vi "Road.vi"(1 "Road Width":i8, 2 "coordinate":T1, 3 "Map in":bool[][](array[boolean])) -> (0 "Map out":bool[][](array[boolean]))   [LabVIEW 2020]
uses:
  <vilib>/numeric/Random Number (Range) I64.vi
  <vilib>/numeric/sub_Random U32.vi
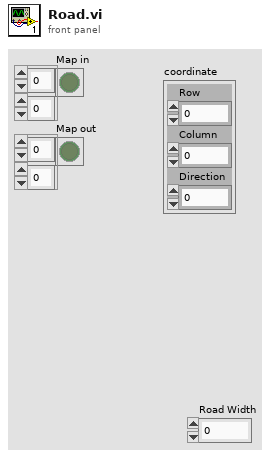
[diagram p1: front panel]
types:
  T1 = cluster{"Row":i32, "Column":i32, "Direction":i32}
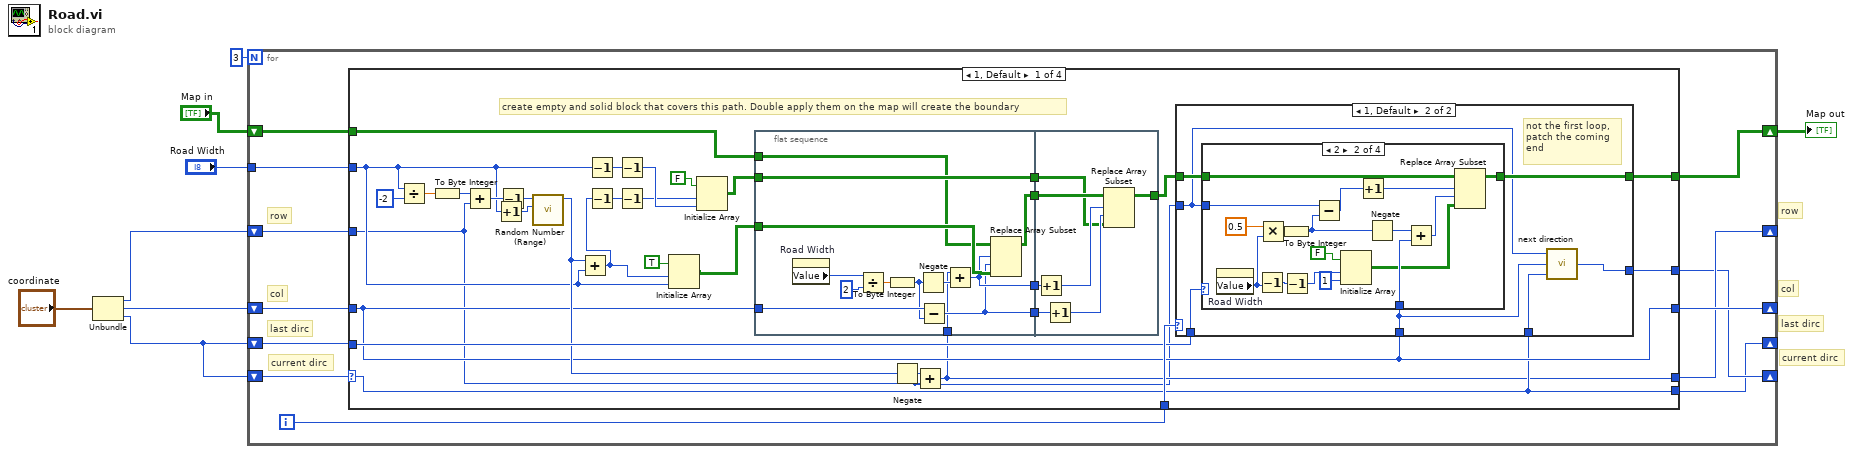
[diagram p0: block diagram]
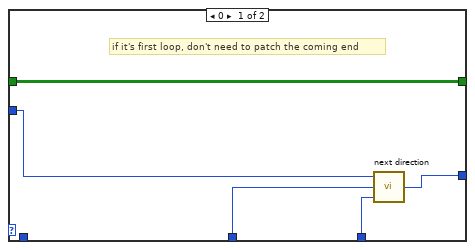
[diagram p2: hidden frame]
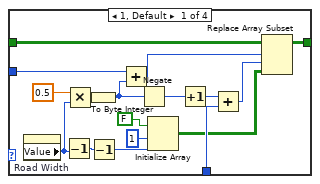
[diagram p3: hidden frame]
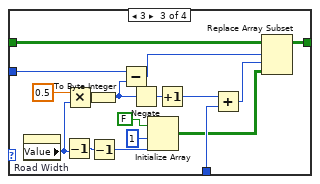
[diagram p4: hidden frame]
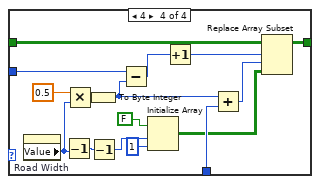
[diagram p5: hidden frame]
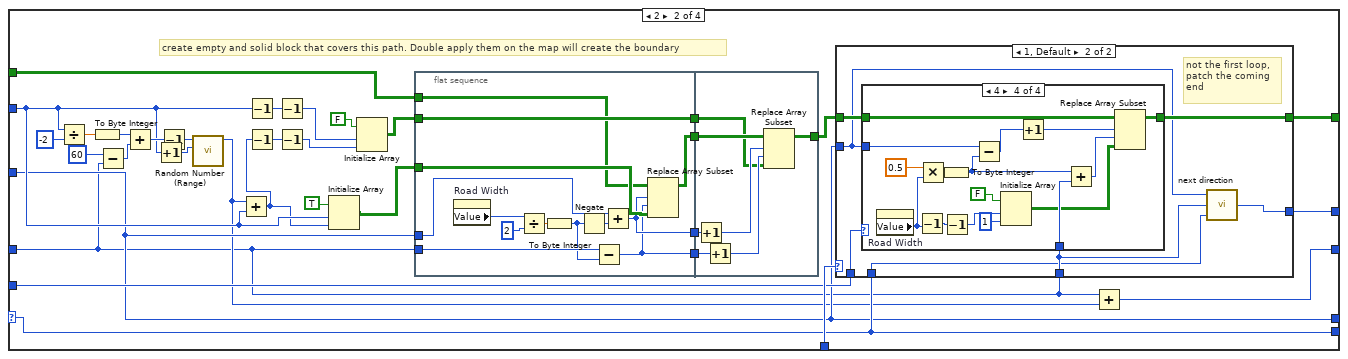
[diagram p6: hidden frame]
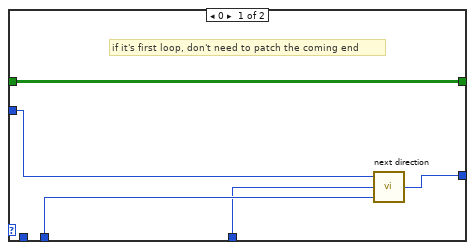
[diagram p7: hidden frame]
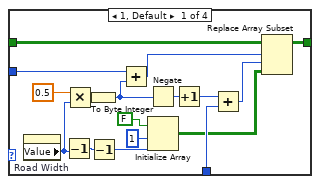
[diagram p8: hidden frame]
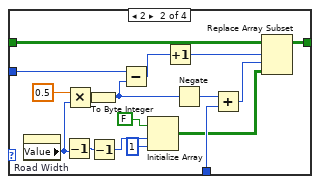
[diagram p9: hidden frame]
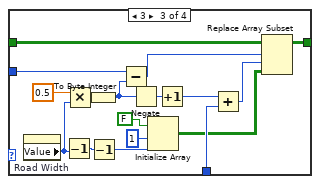
[diagram p10: hidden frame]
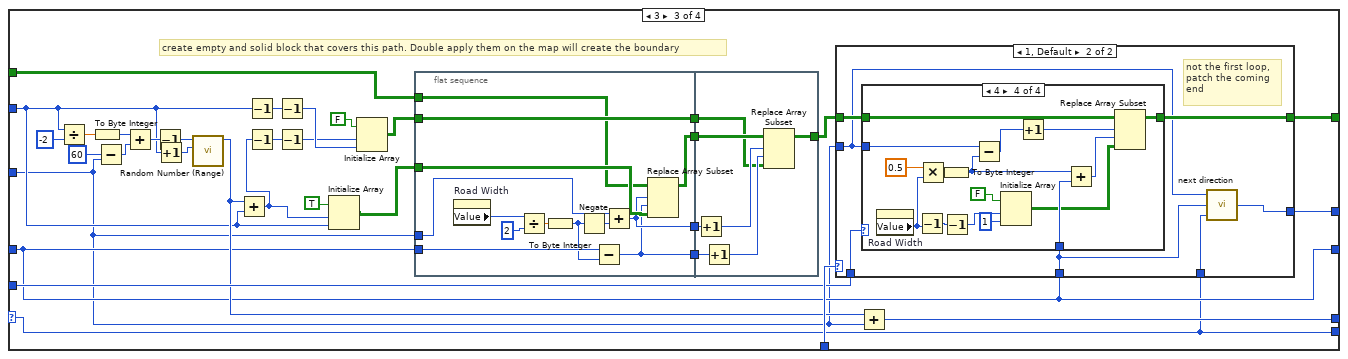
[diagram p11: hidden frame]
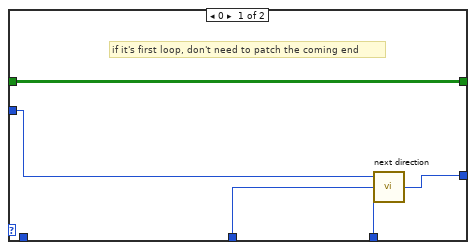
[diagram p12: hidden frame]
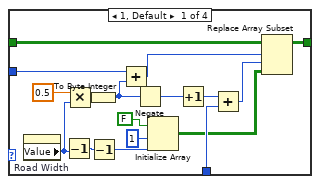
[diagram p13: hidden frame]
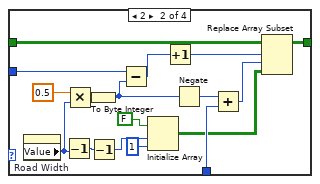
[diagram p14: hidden frame]
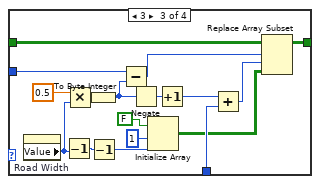
[diagram p15: hidden frame]
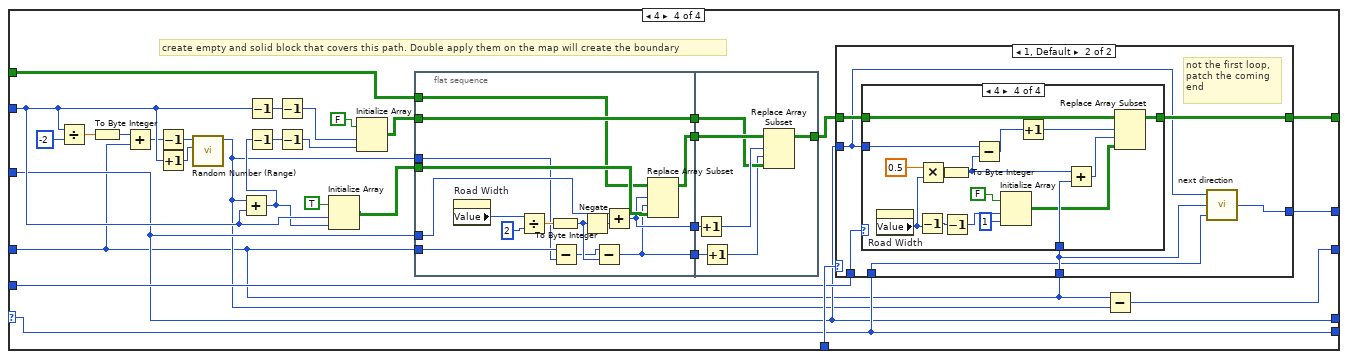
[diagram p16: hidden frame]
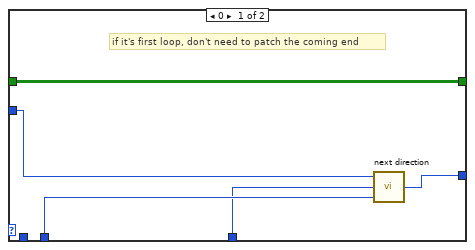
[diagram p17: hidden frame]
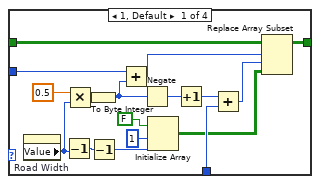
[diagram p18: hidden frame]
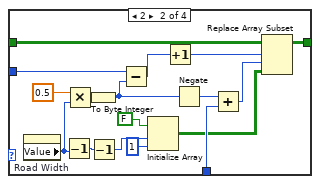
[diagram p19: hidden frame]
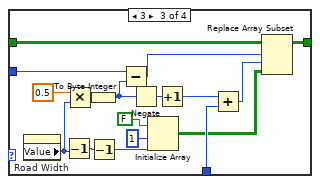
[diagram p20: hidden frame]
diagram:
  # "row"
  # "col"
  # "last dirc"
  # "current dirc"
  n1 = Unbundle("coordinate") -> ("Row"=w3:i32, "Column"=w2:i32, "Direction"=w1:i32)
  n2 = for {
    N: 3 -> [_]
    tunnel: "Road Width" -> [w19]
    shift-right: [w12] -> _
    shift-left: w1 -> [w20]
    shift-right: [w11] -> _
    shift-left: w1 -> [w14]
    shift-right: [w13] -> _
    shift-left: w3 -> [w10]
    shift-right: [w16] -> _
    shift-left: w2 -> [w18]
    shift-right: [w15] -> w5
    shift-left: "Map in" -> [w17]
    i -> [w9]
    # "row"
    # "col"
    # "last dirc"
    # "current dirc"
    n3 = case shown="1, Default" w20 {
      selector: w20 -> [w26 w163 w289 w427]
      tunnel: w19 -> [w30 w158 w294 w424]
      tunnel: w10 -> [w21 w155 w284 w419]
      tunnel: w18 -> [w29 w152 w293 w416]
      tunnel: w17 -> [w31 w166 w295 w430]
      tunnel: w9 -> [w52 w184 w316 w446]
      tunnel: [w22 w155 w292 w419] -> w13
      tunnel: [w29 w154 w293 w418] -> w16
      tunnel: [w51 w183 w315 w445] -> w15
      tunnel: w14 -> [w50 w182 w314 w444]
      tunnel: [w27 w164 w290 w428] -> w12
      tunnel: [w26 w163 w289 w427] -> w11
      frame 1, Default {
        # "create empty and solid block that covers this path. Double apply them on the map will create the boundary"
        n4 = Divide(x=w30, y=i8 -2) -> (x/y=w33:dbl)
        n5 = To Byte Integer(number=w33) -> (8bit integer=w34:i8)
        n6 = Add(x=w34, y=w21) -> (x+y=w35:i64)
        n7 = Increment(x=w30) -> (x+1=w36:i8)
        n8 = Decrement(x=w35) -> (x-1=w23:i64)
        n9 = call-poly <vilib>:"Random Number (Range).vi"("lower bound (-100)"=w36, "upper bound (100)"=w23) -> ("number"=w45:i64)  [unwired: 9 in]
        n10 = Add(x=w45, y=w30) -> (x+y=w24:i64)
        n11 = Decrement(x=w30) -> (x-1=w41:i8)
        n12 = Decrement(x=w24) -> (x-1=w39:i64)
        n13 = Decrement(x=w41) -> (x-1=w42:i8)
        n14 = Decrement(x=w39) -> (x-1=w40:i64)
        n15 = Initialize Array(TRUE, w24, w30) -> (w43:bool[][])
        n16 = Initialize Array(FALSE, w40, w42) -> (w44:bool[][])
        n17 = flat-sequence {
          tunnel: w29 -> [w63]
          tunnel: [w61] -> w49
          tunnel: w43 -> [w60]
          tunnel: [w59] -> w48
          tunnel: [w58] -> w47
          tunnel: w44 -> [w57]
          tunnel: [w57] -> w46
          tunnel: w31 -> [w56]
          tunnel: w22 -> [w53]
          tunnel: w49 -> [w72]
          tunnel: w48 -> [w71]
          tunnel: w47 -> [w69]
          tunnel: w46 -> [w67]
          tunnel: [w66] -> w28
          frame #0 {
            n18 = property on="Road Width" class="DigNum (strict)"() -> ("Value"=w55:i8)  [unwired: 2 in, 2 out]
            n19 = Divide(x=w55, y=i8 2) -> (x/y=w64:dbl)
            n20 = To Byte Integer(number=w64) -> (8bit integer=w62:i8)
            n21 = Negate(x=w62) -> (-x=w54:i8)
            n22 = Subtract(x=w63, y=w62) -> (x-y=w58:i64)
            n23 = Add(x=w53, y=w54) -> (x+y=w59:i64)
            n24 = Replace Array Subset(array=w56, new element=w60, index (row)=w59, index (col)=w58) -> (w61:bool[][])
          }
          frame #1 {
            n25 = Increment(x=w71) -> (x+1=w70:i64)
            n26 = Increment(x=w69) -> (x+1=w68:i64)
            n27 = Replace Array Subset(array=w72, new element=w67, index (row)=w70, index (col)=w68) -> (w66:bool[][])
          }
        }
        n28 = Negate(x=w45) -> (-x=w25:i64)
        n29 = Add(x=w25, y=w21) -> (x+y=w22:i64)
        n30 = case shown="1, Default" w52 {
          tunnel: [w77 w83] -> w51
          tunnel: w50 -> [_ w84]
          tunnel: w21 -> [w73 w81]
          tunnel: w29 -> [w75 w79]
          tunnel: w28 -> [w77 w82]
          tunnel: w26 -> [w76 w78]
          tunnel: [w74 w80] -> w27
          frame 0 {
            # "if it's first loop, don't need to patch the coming end"
            n31 = call "next direction.vi"("current direc"=w76, "col"=w75, "row"=w73) -> ("next direc"=w74:i32)
          }
          frame 1, Default {
            # "not the first loop,\npatch the coming\nend"
            n32 = case shown="2" w84 {
              tunnel: w81 -> [w94 w113 w128 w146]
              tunnel: w79 -> [w90 w111 w124 w144]
              tunnel: [w87 w108 w121 w141] -> w83
              tunnel: w82 -> [w86 w102 w119 w136]
              frame 1, Default {
                n33 = property on="Road Width" class="DigNum (strict)"() -> ("Value"=w96:i8)  [unwired: 2 in, 2 out]
                n34 = Decrement(x=w96) -> (x-1=w100:i8)
                n35 = Multiply(x=0.5, y=w96) -> (x*y=w95:dbl)
                n36 = To Byte Integer(number=w95) -> (8bit integer=w92:i8)
                n37 = Decrement(x=w100) -> (x-1=w99:i8)
                n38 = Add(x=w94, y=w92) -> (x+y=w93:i64)
                n39 = Negate(x=w92) -> (-x=w85:i8)
                n40 = Initialize Array(FALSE, 1 ("dimension size"), w99) -> (w88:bool[][])
                n41 = Increment(x=w85) -> (x+1=w91:i8)
                n42 = Add(x=w91, y=w90) -> (x+y=w89:i64)
                n43 = Replace Array Subset(array=w86, new element=w88, index (row)=w93, index (col)=w89) -> (w87:bool[][])
              }
              frame 2 {
                n44 = property on="Road Width" class="DigNum (strict)"() -> ("Value"=w115:i8)  [unwired: 2 in, 2 out]
                n45 = Decrement(x=w115) -> (x-1=w117:i8)
                n46 = Multiply(x=0.5, y=w115) -> (x*y=w114:dbl)
                n47 = To Byte Integer(number=w114) -> (8bit integer=w104:i8)
                n48 = Decrement(x=w117) -> (x-1=w107:i8)
                n49 = Subtract(x=w113, y=w104) -> (x-y=w112:i64)
                n50 = Initialize Array(FALSE, w107, 1 ("dimension size")) -> (w109:bool[][])
                n51 = Increment(x=w112) -> (x+1=w105:i64)
                n52 = Negate(x=w104) -> (-x=w103:i8)
                n53 = Add(x=w103, y=w111) -> (x+y=w110:i64)
                n54 = Replace Array Subset(array=w102, new element=w109, index (row)=w105, index (col)=w110) -> (w108:bool[][])
              }
              frame 3 {
                n55 = property on="Road Width" class="DigNum (strict)"() -> ("Value"=w130:i8)  [unwired: 2 in, 2 out]
                n56 = Decrement(x=w130) -> (x-1=w134:i8)
                n57 = Multiply(x=0.5, y=w130) -> (x*y=w129:dbl)
                n58 = To Byte Integer(number=w129) -> (8bit integer=w126:i8)
                n59 = Decrement(x=w134) -> (x-1=w133:i8)
                n60 = Subtract(x=w128, y=w126) -> (x-y=w127:i64)
                n61 = Negate(x=w126) -> (-x=w120:i8)
                n62 = Initialize Array(FALSE, 1 ("dimension size"), w133) -> (w122:bool[][])
                n63 = Increment(x=w120) -> (x+1=w125:i8)
                n64 = Add(x=w125, y=w124) -> (x+y=w123:i64)
                n65 = Replace Array Subset(array=w119, new element=w122, index (row)=w127, index (col)=w123) -> (w121:bool[][])
              }
              frame 4 {
                n66 = property on="Road Width" class="DigNum (strict)"() -> ("Value"=w148:i8)  [unwired: 2 in, 2 out]
                n67 = Decrement(x=w148) -> (x-1=w150:i8)
                n68 = Multiply(x=0.5, y=w148) -> (x*y=w147:dbl)
                n69 = To Byte Integer(number=w147) -> (8bit integer=w137:i8)
                n70 = Decrement(x=w150) -> (x-1=w140:i8)
                n71 = Subtract(x=w146, y=w137) -> (x-y=w145:i64)
                n72 = Initialize Array(FALSE, w140, 1 ("dimension size")) -> (w142:bool[][])
                n73 = Increment(x=w145) -> (x+1=w138:i64)
                n74 = Add(x=w137, y=w144) -> (x+y=w143:i64)
                n75 = Replace Array Subset(array=w136, new element=w142, index (row)=w138, index (col)=w143) -> (w141:bool[][])
              }
            }
            n76 = call "next direction.vi"("current direc"=w78, "col"=w79, "row"=w81) -> ("next direc"=w80:i32)
          }
        }
      }
      frame 2 {
        # "create empty and solid block that covers this path. Double apply them on the map will create the boundary"
        n77 = Divide(x=w158, y=i8 -2) -> (x/y=w168:dbl)
        n78 = To Byte Integer(number=w168) -> (8bit integer=w169:i8)
        n79 = Subtract(x=i8 60, y=w152) -> (x-y=w161:i64)
        n80 = Add(x=w169, y=w161) -> (x+y=w170:i64)
        n81 = Increment(x=w158) -> (x+1=w171:i8)
        n82 = Decrement(x=w170) -> (x-1=w156:i64)
        n83 = call-poly <vilib>:"Random Number (Range).vi"("lower bound (-100)"=w171, "upper bound (100)"=w156) -> ("number"=w153:i64)  [unwired: 9 in]
        n84 = Add(x=w153, y=w158) -> (x+y=w157:i64)
        n85 = Decrement(x=w158) -> (x-1=w175:i8)
        n86 = Decrement(x=w157) -> (x-1=w174:i64)
        n87 = Decrement(x=w175) -> (x-1=w160:i8)
        n88 = Decrement(x=w174) -> (x-1=w159:i64)
        n89 = Initialize Array(TRUE, w158, w157) -> (w176:bool[][])
        n90 = Initialize Array(FALSE, w160, w159) -> (w177:bool[][])
        n91 = flat-sequence {
          tunnel: w155 -> [w196]
          tunnel: w152 -> [w194]
          tunnel: [w192] -> w181
          tunnel: w176 -> [w191]
          tunnel: [w190] -> w180
          tunnel: [w189] -> w179
          tunnel: w177 -> [w188]
          tunnel: [w188] -> w178
          tunnel: w166 -> [w187]
          tunnel: w181 -> [w204]
          tunnel: w180 -> [w203]
          tunnel: w179 -> [w201]
          tunnel: w178 -> [w199]
          tunnel: [w198] -> w165
          frame #0 {
            n92 = property on="Road Width" class="DigNum (strict)"() -> ("Value"=w186:i8)  [unwired: 2 in, 2 out]
            n93 = Divide(x=w186, y=i8 2) -> (x/y=w195:dbl)
            n94 = To Byte Integer(number=w195) -> (8bit integer=w193:i8)
            n95 = Negate(x=w193) -> (-x=w185:i8)
            n96 = Subtract(x=w194, y=w193) -> (x-y=w189:i64)
            n97 = Add(x=w196, y=w185) -> (x+y=w190:i64)
            n98 = Replace Array Subset(array=w187, new element=w191, index (row)=w190, index (col)=w189) -> (w192:bool[][])
          }
          frame #1 {
            n99 = Increment(x=w203) -> (x+1=w202:i64)
            n100 = Increment(x=w201) -> (x+1=w200:i64)
            n101 = Replace Array Subset(array=w204, new element=w199, index (row)=w202, index (col)=w200) -> (w198:bool[][])
          }
        }
        n102 = case shown="1, Default" w184 {
          tunnel: [w209 w215] -> w183
          tunnel: w182 -> [_ w216]
          tunnel: w155 -> [w205 w213]
          tunnel: w152 -> [w207 w211]
          tunnel: w165 -> [w209 w214]
          tunnel: w163 -> [w208 w210]
          tunnel: [w206 w212] -> w164
          frame 0 {
            # "if it's first loop, don't need to patch the coming end"
            n103 = call "next direction.vi"("current direc"=w208, "col"=w207, "row"=w205) -> ("next direc"=w206:i32)
          }
          frame 1, Default {
            # "not the first loop,\npatch the coming\nend"
            n104 = case shown="4" w216 {
              tunnel: w213 -> [w226 w245 w260 w278]
              tunnel: w211 -> [w222 w243 w256 w276]
              tunnel: [w219 w240 w253 w273] -> w215
              tunnel: w214 -> [w218 w234 w251 w268]
              frame 1, Default {
                n105 = property on="Road Width" class="DigNum (strict)"() -> ("Value"=w228:i8)  [unwired: 2 in, 2 out]
                n106 = Decrement(x=w228) -> (x-1=w232:i8)
                n107 = Multiply(x=0.5, y=w228) -> (x*y=w227:dbl)
                n108 = To Byte Integer(number=w227) -> (8bit integer=w224:i8)
                n109 = Decrement(x=w232) -> (x-1=w231:i8)
                n110 = Add(x=w226, y=w224) -> (x+y=w225:i64)
                n111 = Negate(x=w224) -> (-x=w223:i8)
                n112 = Initialize Array(FALSE, 1 ("dimension size"), w231) -> (w220:bool[][])
                n113 = Increment(x=w223) -> (x+1=w217:i8)
                n114 = Add(x=w217, y=w222) -> (x+y=w221:i64)
                n115 = Replace Array Subset(array=w218, new element=w220, index (row)=w225, index (col)=w221) -> (w219:bool[][])
              }
              frame 2 {
                n116 = property on="Road Width" class="DigNum (strict)"() -> ("Value"=w247:i8)  [unwired: 2 in, 2 out]
                n117 = Decrement(x=w247) -> (x-1=w249:i8)
                n118 = Multiply(x=0.5, y=w247) -> (x*y=w246:dbl)
                n119 = To Byte Integer(number=w246) -> (8bit integer=w236:i8)
                n120 = Decrement(x=w249) -> (x-1=w239:i8)
                n121 = Subtract(x=w245, y=w236) -> (x-y=w244:i64)
                n122 = Initialize Array(FALSE, w239, 1 ("dimension size")) -> (w241:bool[][])
                n123 = Increment(x=w244) -> (x+1=w237:i64)
                n124 = Negate(x=w236) -> (-x=w235:i8)
                n125 = Add(x=w235, y=w243) -> (x+y=w242:i64)
                n126 = Replace Array Subset(array=w234, new element=w241, index (row)=w237, index (col)=w242) -> (w240:bool[][])
              }
              frame 3 {
                n127 = property on="Road Width" class="DigNum (strict)"() -> ("Value"=w262:i8)  [unwired: 2 in, 2 out]
                n128 = Decrement(x=w262) -> (x-1=w266:i8)
                n129 = Multiply(x=0.5, y=w262) -> (x*y=w261:dbl)
                n130 = To Byte Integer(number=w261) -> (8bit integer=w258:i8)
                n131 = Decrement(x=w266) -> (x-1=w265:i8)
                n132 = Subtract(x=w260, y=w258) -> (x-y=w259:i64)
                n133 = Negate(x=w258) -> (-x=w252:i8)
                n134 = Initialize Array(FALSE, 1 ("dimension size"), w265) -> (w254:bool[][])
                n135 = Increment(x=w252) -> (x+1=w257:i8)
                n136 = Add(x=w257, y=w256) -> (x+y=w255:i64)
                n137 = Replace Array Subset(array=w251, new element=w254, index (row)=w259, index (col)=w255) -> (w253:bool[][])
              }
              frame 4 {
                n138 = property on="Road Width" class="DigNum (strict)"() -> ("Value"=w280:i8)  [unwired: 2 in, 2 out]
                n139 = Decrement(x=w280) -> (x-1=w282:i8)
                n140 = Multiply(x=0.5, y=w280) -> (x*y=w279:dbl)
                n141 = To Byte Integer(number=w279) -> (8bit integer=w269:i8)
                n142 = Decrement(x=w282) -> (x-1=w272:i8)
                n143 = Subtract(x=w278, y=w269) -> (x-y=w277:i64)
                n144 = Initialize Array(FALSE, w272, 1 ("dimension size")) -> (w274:bool[][])
                n145 = Increment(x=w277) -> (x+1=w270:i64)
                n146 = Add(x=w269, y=w276) -> (x+y=w275:i64)
                n147 = Replace Array Subset(array=w268, new element=w274, index (row)=w270, index (col)=w275) -> (w273:bool[][])
              }
            }
            n148 = call "next direction.vi"("current direc"=w210, "col"=w211, "row"=w213) -> ("next direc"=w212:i32)
          }
        }
        n149 = Add(x=w152, y=w153) -> (x+y=w154:i64)
      }
      frame 3 {
        # "create empty and solid block that covers this path. Double apply them on the map will create the boundary"
        n150 = Divide(x=w294, y=i8 -2) -> (x/y=w297:dbl)
        n151 = To Byte Integer(number=w297) -> (8bit integer=w298:i8)
        n152 = Subtract(x=i8 60, y=w284) -> (x-y=w285:i64)
        n153 = Add(x=w298, y=w285) -> (x+y=w299:i64)
        n154 = Decrement(x=w299) -> (x-1=w287:i64)
        n155 = Increment(x=w294) -> (x+1=w300:i8)
        n156 = call-poly <vilib>:"Random Number (Range).vi"("lower bound (-100)"=w300, "upper bound (100)"=w287) -> ("number"=w309:i64)  [unwired: 9 in]
        n157 = Add(x=w309, y=w294) -> (x+y=w288:i64)
        n158 = Decrement(x=w294) -> (x-1=w305:i8)
        n159 = Decrement(x=w288) -> (x-1=w303:i64)
        n160 = Decrement(x=w305) -> (x-1=w306:i8)
        n161 = Decrement(x=w303) -> (x-1=w304:i64)
        n162 = Initialize Array(TRUE, w288, w294) -> (w307:bool[][])
        n163 = Initialize Array(FALSE, w304, w306) -> (w308:bool[][])
        n164 = flat-sequence {
          tunnel: w284 -> [w328]
          tunnel: w293 -> [w326]
          tunnel: [w324] -> w313
          tunnel: w307 -> [w323]
          tunnel: [w322] -> w312
          tunnel: [w321] -> w311
          tunnel: w308 -> [w320]
          tunnel: [w320] -> w310
          tunnel: w295 -> [w319]
          tunnel: w313 -> [w336]
          tunnel: w312 -> [w335]
          tunnel: w311 -> [w333]
          tunnel: w310 -> [w331]
          tunnel: [w330] -> w291
          frame #0 {
            n165 = property on="Road Width" class="DigNum (strict)"() -> ("Value"=w318:i8)  [unwired: 2 in, 2 out]
            n166 = Divide(x=w318, y=i8 2) -> (x/y=w327:dbl)
            n167 = To Byte Integer(number=w327) -> (8bit integer=w325:i8)
            n168 = Negate(x=w325) -> (-x=w317:i8)
            n169 = Subtract(x=w326, y=w325) -> (x-y=w321:i64)
            n170 = Add(x=w328, y=w317) -> (x+y=w322:i64)
            n171 = Replace Array Subset(array=w319, new element=w323, index (row)=w322, index (col)=w321) -> (w324:bool[][])
          }
          frame #1 {
            n172 = Increment(x=w335) -> (x+1=w334:i64)
            n173 = Increment(x=w333) -> (x+1=w332:i64)
            n174 = Replace Array Subset(array=w336, new element=w331, index (row)=w334, index (col)=w332) -> (w330:bool[][])
          }
        }
        n175 = case shown="1, Default" w316 {
          tunnel: [w341 w347] -> w315
          tunnel: w314 -> [_ w348]
          tunnel: w284 -> [w337 w345]
          tunnel: w293 -> [w339 w343]
          tunnel: w291 -> [w341 w346]
          tunnel: w289 -> [w340 w342]
          tunnel: [w338 w344] -> w290
          frame 0 {
            # "if it's first loop, don't need to patch the coming end"
            n176 = call "next direction.vi"("current direc"=w340, "col"=w339, "row"=w337) -> ("next direc"=w338:i32)
          }
          frame 1, Default {
            # "not the first loop,\npatch the coming\nend"
            n177 = case shown="4" w348 {
              tunnel: w345 -> [w358 w377 w392 w410]
              tunnel: w343 -> [w354 w375 w388 w408]
              tunnel: [w351 w372 w385 w405] -> w347
              tunnel: w346 -> [w350 w366 w383 w400]
              frame 1, Default {
                n178 = property on="Road Width" class="DigNum (strict)"() -> ("Value"=w360:i8)  [unwired: 2 in, 2 out]
                n179 = Decrement(x=w360) -> (x-1=w364:i8)
                n180 = Multiply(x=0.5, y=w360) -> (x*y=w359:dbl)
                n181 = To Byte Integer(number=w359) -> (8bit integer=w356:i8)
                n182 = Decrement(x=w364) -> (x-1=w363:i8)
                n183 = Add(x=w358, y=w356) -> (x+y=w357:i64)
                n184 = Negate(x=w356) -> (-x=w349:i8)
                n185 = Initialize Array(FALSE, 1 ("dimension size"), w363) -> (w352:bool[][])
                n186 = Increment(x=w349) -> (x+1=w355:i8)
                n187 = Add(x=w355, y=w354) -> (x+y=w353:i64)
                n188 = Replace Array Subset(array=w350, new element=w352, index (row)=w357, index (col)=w353) -> (w351:bool[][])
              }
              frame 2 {
                n189 = property on="Road Width" class="DigNum (strict)"() -> ("Value"=w379:i8)  [unwired: 2 in, 2 out]
                n190 = Decrement(x=w379) -> (x-1=w381:i8)
                n191 = Multiply(x=0.5, y=w379) -> (x*y=w378:dbl)
                n192 = To Byte Integer(number=w378) -> (8bit integer=w368:i8)
                n193 = Decrement(x=w381) -> (x-1=w371:i8)
                n194 = Subtract(x=w377, y=w368) -> (x-y=w376:i64)
                n195 = Initialize Array(FALSE, w371, 1 ("dimension size")) -> (w373:bool[][])
                n196 = Increment(x=w376) -> (x+1=w369:i64)
                n197 = Negate(x=w368) -> (-x=w367:i8)
                n198 = Add(x=w367, y=w375) -> (x+y=w374:i64)
                n199 = Replace Array Subset(array=w366, new element=w373, index (row)=w369, index (col)=w374) -> (w372:bool[][])
              }
              frame 3 {
                n200 = property on="Road Width" class="DigNum (strict)"() -> ("Value"=w394:i8)  [unwired: 2 in, 2 out]
                n201 = Decrement(x=w394) -> (x-1=w398:i8)
                n202 = Multiply(x=0.5, y=w394) -> (x*y=w393:dbl)
                n203 = To Byte Integer(number=w393) -> (8bit integer=w390:i8)
                n204 = Decrement(x=w398) -> (x-1=w397:i8)
                n205 = Subtract(x=w392, y=w390) -> (x-y=w391:i64)
                n206 = Negate(x=w390) -> (-x=w384:i8)
                n207 = Initialize Array(FALSE, 1 ("dimension size"), w397) -> (w386:bool[][])
                n208 = Increment(x=w384) -> (x+1=w389:i8)
                n209 = Add(x=w389, y=w388) -> (x+y=w387:i64)
                n210 = Replace Array Subset(array=w383, new element=w386, index (row)=w391, index (col)=w387) -> (w385:bool[][])
              }
              frame 4 {
                n211 = property on="Road Width" class="DigNum (strict)"() -> ("Value"=w412:i8)  [unwired: 2 in, 2 out]
                n212 = Decrement(x=w412) -> (x-1=w414:i8)
                n213 = Multiply(x=0.5, y=w412) -> (x*y=w411:dbl)
                n214 = To Byte Integer(number=w411) -> (8bit integer=w401:i8)
                n215 = Decrement(x=w414) -> (x-1=w404:i8)
                n216 = Subtract(x=w410, y=w401) -> (x-y=w409:i64)
                n217 = Initialize Array(FALSE, w404, 1 ("dimension size")) -> (w406:bool[][])
                n218 = Increment(x=w409) -> (x+1=w402:i64)
                n219 = Add(x=w401, y=w408) -> (x+y=w407:i64)
                n220 = Replace Array Subset(array=w400, new element=w406, index (row)=w402, index (col)=w407) -> (w405:bool[][])
              }
            }
            n221 = call "next direction.vi"("current direc"=w342, "col"=w343, "row"=w345) -> ("next direc"=w344:i32)
          }
        }
        n222 = Add(x=w309, y=w284) -> (x+y=w292:i64)
      }
      frame 4 {
        # "create empty and solid block that covers this path. Double apply them on the map will create the boundary"
        n223 = Divide(x=w424, y=i8 -2) -> (x/y=w432:dbl)
        n224 = To Byte Integer(number=w432) -> (8bit integer=w433:i8)
        n225 = Add(x=w433, y=w416) -> (x+y=w421:i64)
        n226 = Decrement(x=w421) -> (x-1=w420:i64)
        n227 = Increment(x=w424) -> (x+1=w434:i8)
        n228 = call-poly <vilib>:"Random Number (Range).vi"("lower bound (-100)"=w434, "upper bound (100)"=w420) -> ("number"=w417:i64)  [unwired: 9 in]
        n229 = Add(x=w417, y=w424) -> (x+y=w422:i64)
        n230 = Decrement(x=w424) -> (x-1=w438:i8)
        n231 = Decrement(x=w422) -> (x-1=w437:i64)
        n232 = Decrement(x=w438) -> (x-1=w426:i8)
        n233 = Decrement(x=w437) -> (x-1=w425:i64)
        n234 = Initialize Array(TRUE, w424, w422) -> (w439:bool[][])
        n235 = Initialize Array(FALSE, w426, w425) -> (w440:bool[][])
        n236 = flat-sequence {
          tunnel: w419 -> [w460]
          tunnel: w416 -> [w449]
          tunnel: [w457] -> w443
          tunnel: w439 -> [w456]
          tunnel: [w455] -> w442
          tunnel: w440 -> [w454]
          tunnel: [w454] -> w441
          tunnel: w430 -> [w453]
          tunnel: [w451] -> w423
          tunnel: w417 -> [w448]
          tunnel: w443 -> [w468]
          tunnel: w442 -> [w467]
          tunnel: w441 -> [w465]
          tunnel: [w464] -> w429
          tunnel: w423 -> [w463]
          frame #0 {
            n237 = property on="Road Width" class="DigNum (strict)"() -> ("Value"=w452:i8)  [unwired: 2 in, 2 out]
            n238 = Divide(x=w452, y=i8 2) -> (x/y=w459:dbl)
            n239 = To Byte Integer(number=w459) -> (8bit integer=w458:i8)
            n240 = Subtract(x=w449, y=w448) -> (x-y=w450:i64)
            n241 = Negate(x=w458) -> (-x=w447:i8)
            n242 = Subtract(x=w450, y=w458) -> (x-y=w451:i64)
            n243 = Add(x=w460, y=w447) -> (x+y=w455:i64)
            n244 = Replace Array Subset(array=w453, new element=w456, index (row)=w455, index (col)=w451) -> (w457:bool[][])
          }
          frame #1 {
            n245 = Increment(x=w467) -> (x+1=w466:i64)
            n246 = Increment(x=w463) -> (x+1=w462:i64)
            n247 = Replace Array Subset(array=w468, new element=w465, index (row)=w466, index (col)=w462) -> (w464:bool[][])
          }
        }
        n248 = case shown="1, Default" w446 {
          tunnel: [w473 w479] -> w445
          tunnel: w444 -> [_ w480]
          tunnel: w419 -> [w469 w477]
          tunnel: w416 -> [w471 w475]
          tunnel: w429 -> [w473 w478]
          tunnel: w427 -> [w472 w474]
          tunnel: [w470 w476] -> w428
          frame 0 {
            # "if it's first loop, don't need to patch the coming end"
            n249 = call "next direction.vi"("current direc"=w472, "col"=w471, "row"=w469) -> ("next direc"=w470:i32)
          }
          frame 1, Default {
            # "not the first loop,\npatch the coming\nend"
            n250 = case shown="4" w480 {
              tunnel: w477 -> [w490 w509 w524 w542]
              tunnel: w475 -> [w486 w507 w520 w540]
              tunnel: [w483 w504 w517 w537] -> w479
              tunnel: w478 -> [w482 w498 w515 w532]
              frame 1, Default {
                n251 = property on="Road Width" class="DigNum (strict)"() -> ("Value"=w492:i8)  [unwired: 2 in, 2 out]
                n252 = Decrement(x=w492) -> (x-1=w496:i8)
                n253 = Multiply(x=0.5, y=w492) -> (x*y=w491:dbl)
                n254 = To Byte Integer(number=w491) -> (8bit integer=w488:i8)
                n255 = Decrement(x=w496) -> (x-1=w495:i8)
                n256 = Add(x=w490, y=w488) -> (x+y=w489:i64)
                n257 = Negate(x=w488) -> (-x=w481:i8)
                n258 = Initialize Array(FALSE, 1 ("dimension size"), w495) -> (w484:bool[][])
                n259 = Increment(x=w481) -> (x+1=w487:i8)
                n260 = Add(x=w487, y=w486) -> (x+y=w485:i64)
                n261 = Replace Array Subset(array=w482, new element=w484, index (row)=w489, index (col)=w485) -> (w483:bool[][])
              }
              frame 2 {
                n262 = property on="Road Width" class="DigNum (strict)"() -> ("Value"=w511:i8)  [unwired: 2 in, 2 out]
                n263 = Decrement(x=w511) -> (x-1=w513:i8)
                n264 = Multiply(x=0.5, y=w511) -> (x*y=w510:dbl)
                n265 = To Byte Integer(number=w510) -> (8bit integer=w500:i8)
                n266 = Decrement(x=w513) -> (x-1=w503:i8)
                n267 = Subtract(x=w509, y=w500) -> (x-y=w508:i64)
                n268 = Initialize Array(FALSE, w503, 1 ("dimension size")) -> (w505:bool[][])
                n269 = Increment(x=w508) -> (x+1=w501:i64)
                n270 = Negate(x=w500) -> (-x=w499:i8)
                n271 = Add(x=w499, y=w507) -> (x+y=w506:i64)
                n272 = Replace Array Subset(array=w498, new element=w505, index (row)=w501, index (col)=w506) -> (w504:bool[][])
              }
              frame 3 {
                n273 = property on="Road Width" class="DigNum (strict)"() -> ("Value"=w526:i8)  [unwired: 2 in, 2 out]
                n274 = Decrement(x=w526) -> (x-1=w530:i8)
                n275 = Multiply(x=0.5, y=w526) -> (x*y=w525:dbl)
                n276 = To Byte Integer(number=w525) -> (8bit integer=w522:i8)
                n277 = Decrement(x=w530) -> (x-1=w529:i8)
                n278 = Subtract(x=w524, y=w522) -> (x-y=w523:i64)
                n279 = Negate(x=w522) -> (-x=w516:i8)
                n280 = Initialize Array(FALSE, 1 ("dimension size"), w529) -> (w518:bool[][])
                n281 = Increment(x=w516) -> (x+1=w521:i8)
                n282 = Add(x=w521, y=w520) -> (x+y=w519:i64)
                n283 = Replace Array Subset(array=w515, new element=w518, index (row)=w523, index (col)=w519) -> (w517:bool[][])
              }
              frame 4 {
                n284 = property on="Road Width" class="DigNum (strict)"() -> ("Value"=w544:i8)  [unwired: 2 in, 2 out]
                n285 = Decrement(x=w544) -> (x-1=w546:i8)
                n286 = Multiply(x=0.5, y=w544) -> (x*y=w543:dbl)
                n287 = To Byte Integer(number=w543) -> (8bit integer=w533:i8)
                n288 = Decrement(x=w546) -> (x-1=w536:i8)
                n289 = Subtract(x=w542, y=w533) -> (x-y=w541:i64)
                n290 = Initialize Array(FALSE, w536, 1 ("dimension size")) -> (w538:bool[][])
                n291 = Increment(x=w541) -> (x+1=w534:i64)
                n292 = Add(x=w533, y=w540) -> (x+y=w539:i64)
                n293 = Replace Array Subset(array=w532, new element=w538, index (row)=w534, index (col)=w539) -> (w537:bool[][])
              }
            }
            n294 = call "next direction.vi"("current direc"=w474, "col"=w475, "row"=w477) -> ("next direc"=w476:i32)
          }
        }
        n295 = Subtract(x=w416, y=w417) -> (x-y=w418:i64)
      }
    }
  }
  "Map out" <- w5
